vi "ring array.vi"() -> ()   [LabVIEW 2024]
panel:
  out "ring":u16[][](array[ring])
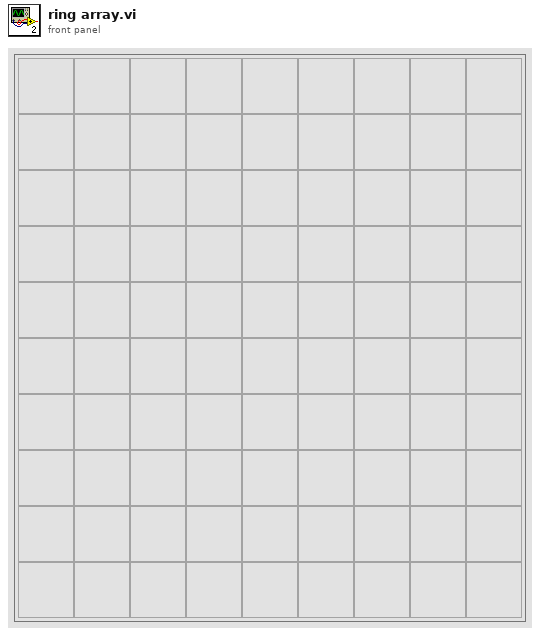
[diagram p1: front panel]
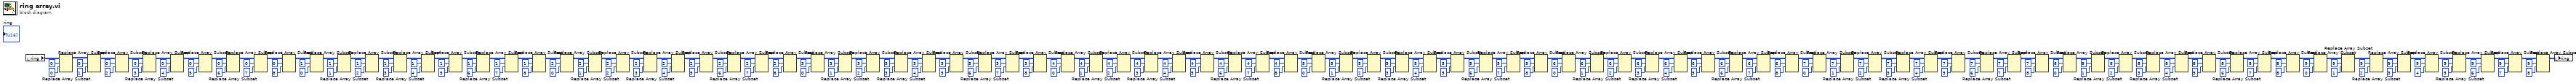
[diagram p0: block diagram]
diagram:
  n1 = local read "ring"() -> (w1:u16[][])
  n2 = Replace Array Subset(array=w1, index (row)=0, index (col)=0) -> (w182:u16[][])  [unwired: 1 in]
  n3 = Replace Array Subset(array=w182, index (row)=0, index (col)=1) -> (w183:u16[][])  [unwired: 1 in]
  n4 = Replace Array Subset(array=w183, index (row)=0, index (col)=2) -> (w184:u16[][])  [unwired: 1 in]
  n5 = Replace Array Subset(array=w184, index (row)=0, index (col)=3) -> (w185:u16[][])  [unwired: 1 in]
  n6 = Replace Array Subset(array=w185, index (row)=0, index (col)=4) -> (w186:u16[][])  [unwired: 1 in]
  n7 = Replace Array Subset(array=w186, index (row)=0, index (col)=5) -> (w187:u16[][])  [unwired: 1 in]
  n8 = Replace Array Subset(array=w187, index (row)=0, index (col)=6) -> (w188:u16[][])  [unwired: 1 in]
  n9 = Replace Array Subset(array=w188, index (row)=0, index (col)=7) -> (w189:u16[][])  [unwired: 1 in]
  n10 = Replace Array Subset(array=w189, index (row)=0, index (col)=8) -> (w190:u16[][])  [unwired: 1 in]
  n11 = Replace Array Subset(array=w190, index (row)=1, index (col)=0) -> (w191:u16[][])  [unwired: 1 in]
  n12 = Replace Array Subset(array=w191, index (row)=1, index (col)=1) -> (w192:u16[][])  [unwired: 1 in]
  n13 = Replace Array Subset(array=w192, index (row)=1, index (col)=2) -> (w193:u16[][])  [unwired: 1 in]
  n14 = Replace Array Subset(array=w193, index (row)=1, index (col)=3) -> (w194:u16[][])  [unwired: 1 in]
  n15 = Replace Array Subset(array=w194, index (row)=1, index (col)=4) -> (w195:u16[][])  [unwired: 1 in]
  n16 = Replace Array Subset(array=w195, index (row)=1, index (col)=5) -> (w196:u16[][])  [unwired: 1 in]
  n17 = Replace Array Subset(array=w196, index (row)=1, index (col)=6) -> (w197:u16[][])  [unwired: 1 in]
  n18 = Replace Array Subset(array=w197, index (row)=1, index (col)=7) -> (w198:u16[][])  [unwired: 1 in]
  n19 = Replace Array Subset(array=w198, index (row)=1, index (col)=8) -> (w199:u16[][])  [unwired: 1 in]
  n20 = Replace Array Subset(array=w199, index (row)=2, index (col)=0) -> (w200:u16[][])  [unwired: 1 in]
  n21 = Replace Array Subset(array=w200, index (row)=2, index (col)=1) -> (w201:u16[][])  [unwired: 1 in]
  n22 = Replace Array Subset(array=w201, index (row)=2, index (col)=2) -> (w202:u16[][])  [unwired: 1 in]
  n23 = Replace Array Subset(array=w202, index (row)=2, index (col)=3) -> (w203:u16[][])  [unwired: 1 in]
  n24 = Replace Array Subset(array=w203, index (row)=2, index (col)=4) -> (w204:u16[][])  [unwired: 1 in]
  n25 = Replace Array Subset(array=w204, index (row)=2, index (col)=5) -> (w205:u16[][])  [unwired: 1 in]
  n26 = Replace Array Subset(array=w205, index (row)=2, index (col)=6) -> (w206:u16[][])  [unwired: 1 in]
  n27 = Replace Array Subset(array=w206, index (row)=2, index (col)=7) -> (w207:u16[][])  [unwired: 1 in]
  n28 = Replace Array Subset(array=w207, index (row)=2, index (col)=8) -> (w208:u16[][])  [unwired: 1 in]
  n29 = Replace Array Subset(array=w208, index (row)=3, index (col)=0) -> (w209:u16[][])  [unwired: 1 in]
  n30 = Replace Array Subset(array=w209, index (row)=3, index (col)=1) -> (w210:u16[][])  [unwired: 1 in]
  n31 = Replace Array Subset(array=w210, index (row)=3, index (col)=2) -> (w211:u16[][])  [unwired: 1 in]
  n32 = Replace Array Subset(array=w211, index (row)=3, index (col)=3) -> (w212:u16[][])  [unwired: 1 in]
  n33 = Replace Array Subset(array=w212, index (row)=3, index (col)=4) -> (w213:u16[][])  [unwired: 1 in]
  n34 = Replace Array Subset(array=w213, index (row)=3, index (col)=5) -> (w214:u16[][])  [unwired: 1 in]
  n35 = Replace Array Subset(array=w214, index (row)=3, index (col)=6) -> (w215:u16[][])  [unwired: 1 in]
  n36 = Replace Array Subset(array=w215, index (row)=3, index (col)=7) -> (w216:u16[][])  [unwired: 1 in]
  n37 = Replace Array Subset(array=w216, index (row)=3, index (col)=8) -> (w217:u16[][])  [unwired: 1 in]
  n38 = Replace Array Subset(array=w217, index (row)=4, index (col)=0) -> (w218:u16[][])  [unwired: 1 in]
  n39 = Replace Array Subset(array=w218, index (row)=4, index (col)=1) -> (w219:u16[][])  [unwired: 1 in]
  n40 = Replace Array Subset(array=w219, index (row)=4, index (col)=2) -> (w220:u16[][])  [unwired: 1 in]
  n41 = Replace Array Subset(array=w220, index (row)=4, index (col)=3) -> (w221:u16[][])  [unwired: 1 in]
  n42 = Replace Array Subset(array=w221, index (row)=4, index (col)=4) -> (w222:u16[][])  [unwired: 1 in]
  n43 = Replace Array Subset(array=w222, index (row)=4, index (col)=5) -> (w223:u16[][])  [unwired: 1 in]
  n44 = Replace Array Subset(array=w223, index (row)=4, index (col)=6) -> (w224:u16[][])  [unwired: 1 in]
  n45 = Replace Array Subset(array=w224, index (row)=4, index (col)=7) -> (w225:u16[][])  [unwired: 1 in]
  n46 = Replace Array Subset(array=w225, index (row)=4, index (col)=8) -> (w226:u16[][])  [unwired: 1 in]
  n47 = Replace Array Subset(array=w226, index (row)=5, index (col)=0) -> (w227:u16[][])  [unwired: 1 in]
  n48 = Replace Array Subset(array=w227, index (row)=5, index (col)=1) -> (w228:u16[][])  [unwired: 1 in]
  n49 = Replace Array Subset(array=w228, index (row)=5, index (col)=2) -> (w229:u16[][])  [unwired: 1 in]
  n50 = Replace Array Subset(array=w229, index (row)=5, index (col)=3) -> (w230:u16[][])  [unwired: 1 in]
  n51 = Replace Array Subset(array=w230, index (row)=5, index (col)=4) -> (w231:u16[][])  [unwired: 1 in]
  n52 = Replace Array Subset(array=w231, index (row)=5, index (col)=5) -> (w232:u16[][])  [unwired: 1 in]
  n53 = Replace Array Subset(array=w232, index (row)=5, index (col)=6) -> (w233:u16[][])  [unwired: 1 in]
  n54 = Replace Array Subset(array=w233, index (row)=5, index (col)=7) -> (w234:u16[][])  [unwired: 1 in]
  n55 = Replace Array Subset(array=w234, index (row)=5, index (col)=8) -> (w235:u16[][])  [unwired: 1 in]
  n56 = Replace Array Subset(array=w235, index (row)=6, index (col)=0) -> (w236:u16[][])  [unwired: 1 in]
  n57 = Replace Array Subset(array=w236, index (row)=6, index (col)=1) -> (w237:u16[][])  [unwired: 1 in]
  n58 = Replace Array Subset(array=w237, index (row)=6, index (col)=2) -> (w238:u16[][])  [unwired: 1 in]
  n59 = Replace Array Subset(array=w238, index (row)=6, index (col)=3) -> (w239:u16[][])  [unwired: 1 in]
  n60 = Replace Array Subset(array=w239, index (row)=6, index (col)=4) -> (w240:u16[][])  [unwired: 1 in]
  n61 = Replace Array Subset(array=w240, index (row)=6, index (col)=5) -> (w241:u16[][])  [unwired: 1 in]
  n62 = Replace Array Subset(array=w241, index (row)=6, index (col)=6) -> (w242:u16[][])  [unwired: 1 in]
  n63 = Replace Array Subset(array=w242, index (row)=6, index (col)=7) -> (w243:u16[][])  [unwired: 1 in]
  n64 = Replace Array Subset(array=w243, index (row)=6, index (col)=8) -> (w244:u16[][])  [unwired: 1 in]
  n65 = Replace Array Subset(array=w244, index (row)=7, index (col)=0) -> (w245:u16[][])  [unwired: 1 in]
  n66 = Replace Array Subset(array=w245, index (row)=7, index (col)=1) -> (w246:u16[][])  [unwired: 1 in]
  n67 = Replace Array Subset(array=w246, index (row)=7, index (col)=2) -> (w247:u16[][])  [unwired: 1 in]
  n68 = Replace Array Subset(array=w247, index (row)=7, index (col)=3) -> (w248:u16[][])  [unwired: 1 in]
  n69 = Replace Array Subset(array=w248, index (row)=7, index (col)=4) -> (w249:u16[][])  [unwired: 1 in]
  n70 = Replace Array Subset(array=w249, index (row)=7, index (col)=5) -> (w250:u16[][])  [unwired: 1 in]
  n71 = Replace Array Subset(array=w250, index (row)=7, index (col)=6) -> (w251:u16[][])  [unwired: 1 in]
  n72 = Replace Array Subset(array=w251, index (row)=7, index (col)=7) -> (w252:u16[][])  [unwired: 1 in]
  n73 = Replace Array Subset(array=w252, index (row)=7, index (col)=8) -> (w253:u16[][])  [unwired: 1 in]
  n74 = Replace Array Subset(array=w253, index (row)=8, index (col)=0) -> (w254:u16[][])  [unwired: 1 in]
  n75 = Replace Array Subset(array=w254, index (row)=8, index (col)=1) -> (w255:u16[][])  [unwired: 1 in]
  n76 = Replace Array Subset(array=w255, index (row)=8, index (col)=2) -> (w256:u16[][])  [unwired: 1 in]
  n77 = Replace Array Subset(array=w256, index (row)=8, index (col)=3) -> (w257:u16[][])  [unwired: 1 in]
  n78 = Replace Array Subset(array=w257, index (row)=8, index (col)=4) -> (w258:u16[][])  [unwired: 1 in]
  n79 = Replace Array Subset(array=w258, index (row)=8, index (col)=5) -> (w259:u16[][])  [unwired: 1 in]
  n80 = Replace Array Subset(array=w259, index (row)=8, index (col)=6) -> (w260:u16[][])  [unwired: 1 in]
  n81 = Replace Array Subset(array=w260, index (row)=8, index (col)=7) -> (w261:u16[][])  [unwired: 1 in]
  n82 = Replace Array Subset(array=w261, index (row)=8, index (col)=8) -> (w262:u16[][])  [unwired: 1 in]
  n83 = Replace Array Subset(array=w262, index (row)=9, index (col)=0) -> (w263:u16[][])  [unwired: 1 in]
  n84 = Replace Array Subset(array=w263, index (row)=9, index (col)=1) -> (w264:u16[][])  [unwired: 1 in]
  n85 = Replace Array Subset(array=w264, index (row)=9, index (col)=2) -> (w265:u16[][])  [unwired: 1 in]
  n86 = Replace Array Subset(array=w265, index (row)=9, index (col)=3) -> (w266:u16[][])  [unwired: 1 in]
  n87 = Replace Array Subset(array=w266, index (row)=9, index (col)=4) -> (w267:u16[][])  [unwired: 1 in]
  n88 = Replace Array Subset(array=w267, index (row)=9, index (col)=5) -> (w268:u16[][])  [unwired: 1 in]
  n89 = Replace Array Subset(array=w268, index (row)=9, index (col)=6) -> (w269:u16[][])  [unwired: 1 in]
  n90 = Replace Array Subset(array=w269, index (row)=9, index (col)=7) -> (w270:u16[][])  [unwired: 1 in]
  n91 = Replace Array Subset(array=w270, index (row)=9, index (col)=8) -> (w271:u16[][])  [unwired: 1 in]
  n92 = local write "ring"(w271) -> ()
